vi "Element Type.vi"(11 "GuiLinkButton in":refnum<class "GuiLinkButton.lvclass">) -> (2 "Element Type":string)   [LabVIEW 2020, in "VolatusGUIElements.lvlib" / "GuiLinkButton.lvclass"]
uses:
  GuiLinkButton.lvclass
  GuiLinkButton.lvclass/GuiLinkButton.ctl
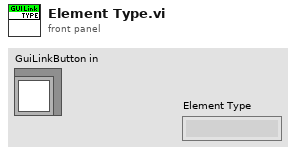
[diagram p1: front panel]
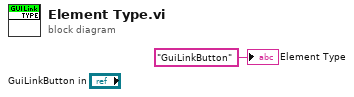
[diagram p0: block diagram]
diagram:
  "Element Type" <- "GuiLinkButton" ("Element Type")
